vi "Initialize.vi"(8 "error in":errorcluster, 11 "4-20mA Settings In":T1) -> (0 "error out":errorcluster, 1 "Initialized":bool, 3 "4-20mA Settings Out":T1)   [LabVIEW 2018, in "Pressure Transmitter Library.lvlib"]
uses:
  Pressure Transmitter Library.lvlib
  Pressure Transmitter Device Settings.ctl
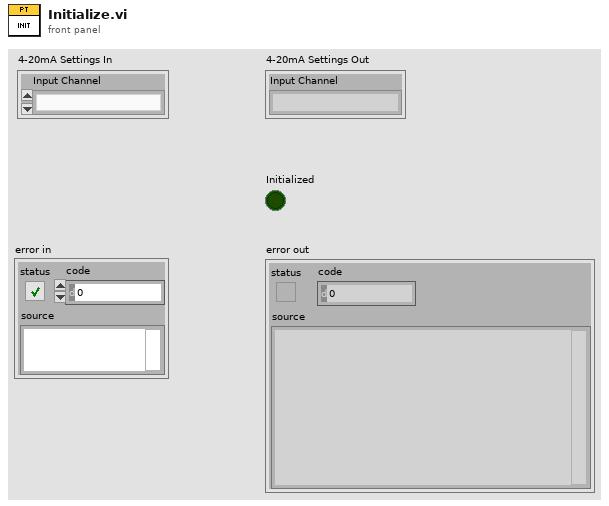
[diagram p1: front panel]
types:
  T1 = typedef "Pressure Transmitter Library.lvlib/Pressure Transmitter Device Settings.ctl" = cluster{"Input Channel ":u16}
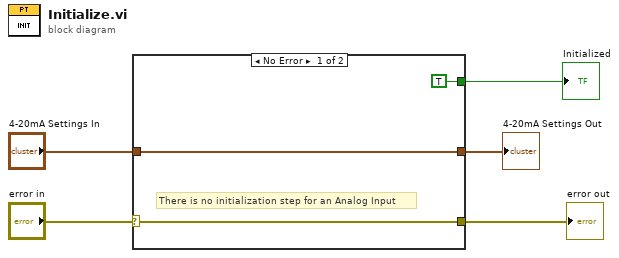
[diagram p0: block diagram]
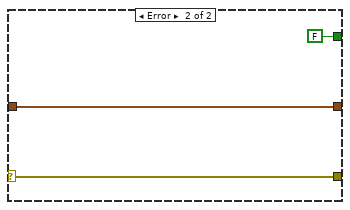
[diagram p2: hidden frame]
diagram:
  n1 = case shown="No Error" "error in" {
    selector: "error in" -> [w8 w10]
    tunnel: [w8 w10] -> w4
    tunnel: "4-20mA Settings In" -> [w7 w11]
    tunnel: [w7 w11] -> w1
    tunnel: [TRUE ("Initialized") FALSE ("Initialized")] -> w3
    frame No Error {
      # "There is no initialization step for an Analog Input"
    }
    frame Error {
    }
  }
  "error out" <- w4
  "Initialized" <- w3
  "4-20mA Settings Out" <- w1
